vi "Move.vi"(8 "error in":errorcluster, 11 "variant in":variant) -> (0 "error out":errorcluster, 3 "variant out":variant, 4 "Voltage out":dbl[](array[numeric]))   [LabVIEW 2013]
uses:
  <vilib>/DAQmx/write.llb/DAQmx Write (Analog 1D DBL NChan 1Samp).vi
  <vilib>/DAQmx/miscellaneous.llb/DAQmx Fill In Error Info.vi
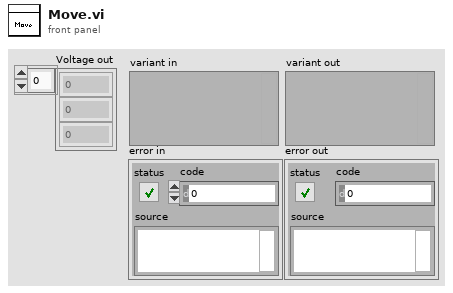
[diagram p1: front panel]
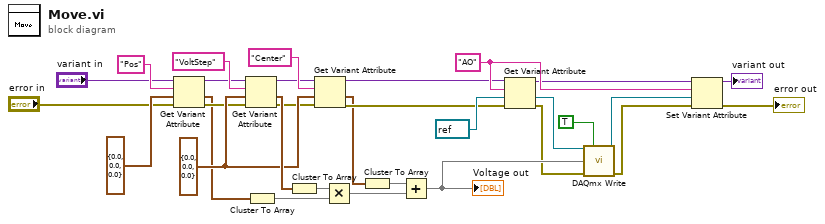
[diagram p0: block diagram]
diagram:
  w31 = "AO" ("name")
  w14 = cluster{"X":dbl, "Y":dbl, "Z":dbl} {"X"=0.0, "Y"=0.0, "Z"=0.0} ("Relative Position")
  n1 = Get Variant Attribute(Variant="variant in", name="Pos", default value (empty Variant)=cluster{"X":dbl, "Y":dbl, "Z":dbl} {"X"=0.0, "Y"=0.0, "Z"=0.0} ("Relative Position"), error in="error in") -> (duplicate Variant=w8:variant, value=w7:cluster{"X":dbl, "Y":dbl, "Z":dbl}, error out=w9:errorcluster)  [unwired: 1 out]
  n2 = Get Variant Attribute(Variant=w8, name="VoltStep", default value (empty Variant)=w14, error in=w9) -> (duplicate Variant=w10:variant, value=w15:cluster{"X":dbl, "Y":dbl, "Z":dbl}, error out=w11:errorcluster)  [unwired: 1 out]
  n3 = Cluster To Array(cluster=w7) -> (array=w18:dbl[])
  n4 = Cluster To Array(cluster=w15) -> (array=w17:dbl[])
  n5 = Get Variant Attribute(Variant=w10, name="Center", default value (empty Variant)=w14, error in=w11) -> (duplicate Variant=w21:variant, value=w16:cluster{"X":dbl, "Y":dbl, "Z":dbl}, error out=w22:errorcluster)  [unwired: 1 out]
  n6 = Multiply(x=w17, y=w18) -> (x*y=w20:dbl[])
  n7 = Cluster To Array(cluster=w16) -> (array=w19:dbl[])
  n8 = Add(x=w19, y=w20) -> (x+y=w26:dbl[])
  "Voltage out" <- w26
  n9 = Get Variant Attribute(Variant=w21, name=w31, default value (empty Variant)=refnum<k21> refnum ("task out"), error in=w22) -> (duplicate Variant=w29:variant, value=w24:refnum<k21>, error out=w25:errorcluster)  [unwired: 1 out]
  n10 = call-poly <vilib>:"DAQmx Write.vi"("task/channels in"=w24, "auto start"=TRUE, "data"=w26, "error in"=w25) -> ("task out"=w30:refnum<k21>, "error out"=w28:errorcluster)  [unwired: 9 in, 1 out]
  n11 = Set Variant Attribute(Variant=w29, name=w31, value=w30, error in=w28) -> (Variant out=→"variant out":variant, error out=→"error out":errorcluster)  [unwired: 1 out]
